vi "多参数测量数据存储.vi"(5 "数据标记表":string(combo)="N", 7 "测量模式":T2(ring)=enum."水样测试", 8 "error in (no error)":errorcluster, 9 "database":string, 10 "table输入":string, 11 "data in":T1) -> (0 "error out":errorcluster)   [LabVIEW 2016, in "斯坦道仪器.lvlib"]
uses:
  <vilib>/Utility/sysdir.llb/System Directory Type.ctl
  <vilib>/addons/database/Connection.llb/DB Tools Open Connec (String).vi
  <vilib>/addons/database/NI_Database_API.lvlib
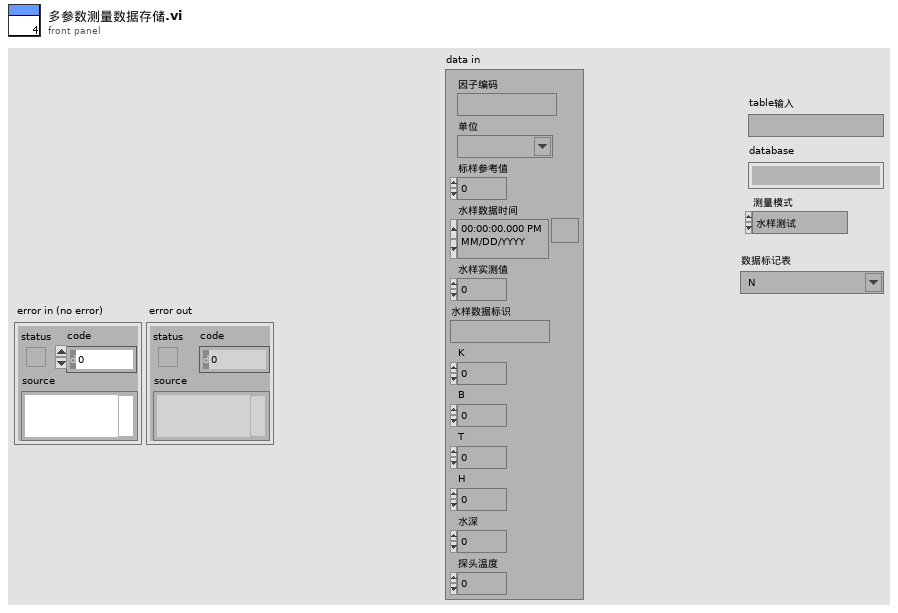
[diagram p1: front panel]
types:
  T1 = cluster{"因子编码":string, "单位":string, "标样参考值":sgl, "水样数据时间":timestamp, "水样实测值":sgl, "水样数据标识":string, "K":sgl, "B":sgl, "T":sgl, "H":sgl, "水深":sgl, "探头温度":sgl}
  T2 = enum16{"待机", "水样测试", "标样核查", "零点核查", "跨度核查", "空白测试", "平行样测试", "加标回收", "空白校准", "标样校准", "初始化（清洗）"}
  T3 = typedef "System Directory Type.ctl" = i32
  T4 = cluster{"时间标识":timestamp, "测量模式":string, "数据类型":string, "监测值":sgl, "单位":string, "数据标识":string, "因子编码":string, "标样参考值":sgl, "K":sgl, "B":sgl, "温度":sgl, "湿度":sgl, "水深":sgl, "探头温度":sgl}
  T5 = typedef "NI_Database_API.lvlib/Conn ObjectReference.ctl" = refnum<k1>
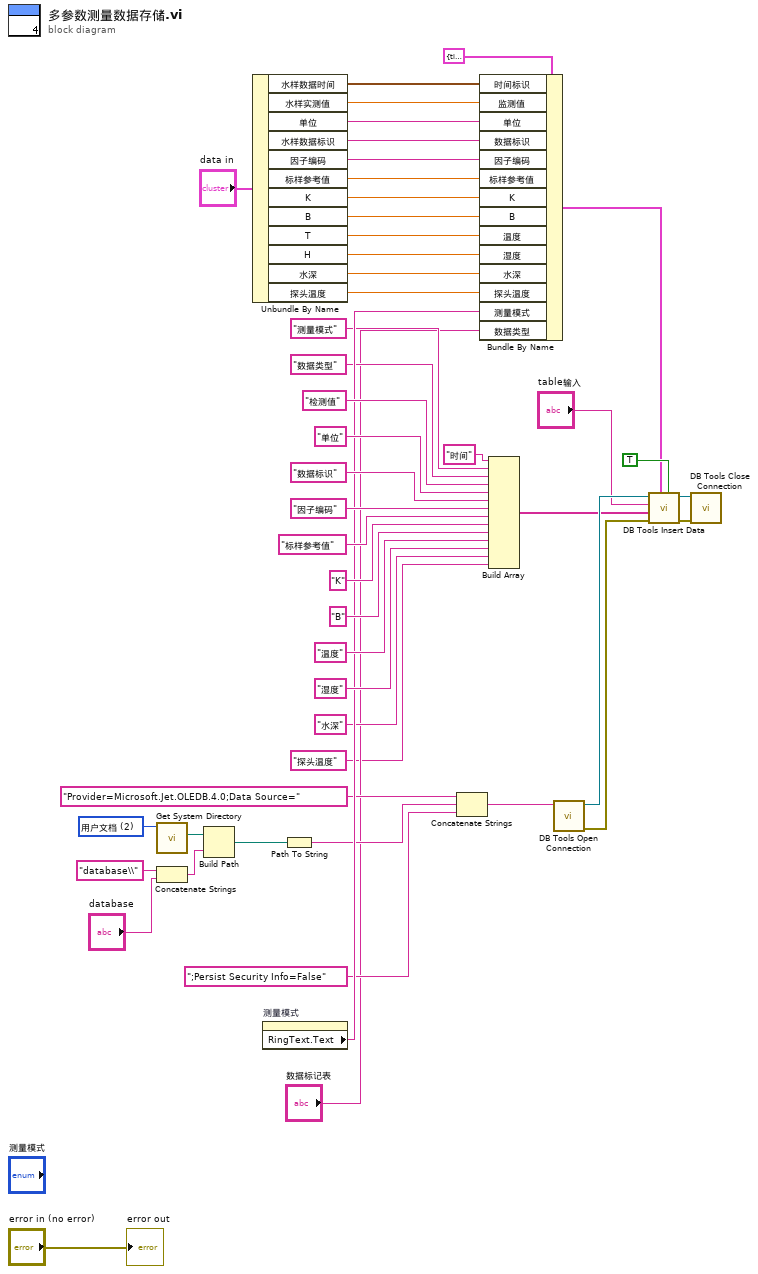
[diagram p0: block diagram]
diagram:
  w21 = T3 2 items=["用户目录"=0, "用户桌面"=1, "用户文档"=2, "用户应用程序数据"=3, "用户设置"=4, "用户临时目录"=5, "公共文档"=6, "公共应用程序数据"=7, "公共设置"=8, "公共缓存"=13, "系统核心库"=9, "系统安装库"=10, "应用程序文件"=11, "启动盘根目录"=12] ("system directory type")
  n1 = call <vilib>:"Get System Directory.vi"("system directory type"=w21) -> ("system directory"=w19:path)  [unwired: 10 in]
  n2 = Concatenate Strings("database\\" ("condition"), "database") -> (w13:string)
  n3 = Build Path(base path=w19, name or relative path=w13) -> (appended path=w18:path)
  n4 = Unbundle By Name("data in") -> ("水样数据时间"=w40:timestamp, "水样实测值"=w39:sgl, "单位"=w31:string, "水样数据标识"=w38:string, "因子编码"=w30:string, "标样参考值"=w32:sgl, "K"=w33:sgl, "B"=w37:sgl, "T"=w36:sgl, "H"=w35:sgl, "水深"=w5:sgl, "探头温度"=w2:sgl)
  n5 = property on="测量模式" class="Enum (严格)"() -> ("RingText.Text"=w29:string)  [unwired: 2 in, 2 out]
  n6 = Path To String(path=w18) -> (string=w17:string)
  n7 = Concatenate Strings("Provider=Microsoft.Jet.OLEDB.4.0;Data Source=" ("condition"), w17, ";Persist Security Info=False" ("condition")) -> (w15:string)
  n8 = Bundle By Name(cluster=T4 {"时间标识"=timestamp(0 s since 1904-01-01), "测量模式"="", "数据类型"="", "监测值"=0.0, "单位"="", "数据标识"="", "因子编码"="", "标样参考值"=0.0, "K"=0.0, "B"=0.0, "温度"=0.0, "湿度"=0.0, "水深"=0.0, "探头温度"=0.0} ("data输出"), "时间标识"=w40, "监测值"=w39, "单位"=w31, "数据标识"=w38, "因子编码"=w30, "标样参考值"=w32, "K"=w33, "B"=w37, "温度"=w36, "湿度"=w35, "水深"=w5, "探头温度"=w2, "测量模式"=w29, "数据类型"="数据标记表") -> (w7:T4)
  n9 = Build Array("时间", "测量模式", "数据类型", "检测值", "单位", "数据标识", "因子编码", "标样参考值", "K", "B", "温度", "湿度", "水深", "探头温度") -> (w8:string[])
  n10 = call-poly <vilib>:"DB Tools Open Connection.vi"("connection information"=w15) -> ("error out"=w10:errorcluster, "connection reference"=w11:T5)  [unwired: 7 in]
  n11 = call <vilib>:"DB Tools Insert Data.vi"("create table? (F)"=TRUE, "data"=w7, "error in (no error)"=w10, "columns"=w8, "table"="table输入", "connection reference"=w11) -> ("error out"=w23:errorcluster, "connection reference out"=w24:T5)  [unwired: 4 in]
  n12 = call <vilib>:"DB Tools Close Connection.vi"("error in (no error)"=w23, "connection reference"=w24) -> ()  [unwired: 5 in, 1 out]
  "error out" <- "error in (no error)"
